vi "OuputMixer5782_1Ghz.vi"(6 "reset":bool, 8 "valid in":bool, 9 "Sine in":fxp<+/-,16,0>[](array[numeric])=[0.0, 0.0, 0.0, 0.0, 0.0, 0.0, 0.0, 0.0], 10 "Cosine in":fxp<+/-,16,0>[](array[numeric])=[0.0, 0.0, 0.0, 0.0, 0.0, 0.0, 0.0, 0.0], 11 "Data in":fxp<+/-,16,14>[](array[numeric])=[0.0, 0.0]) -> (0 "valid out":bool, 3 "test":i16[](array[numeric]))   [LabVIEW 2013]
doc: "Outputs input from channel 0 as I*cos(t)-Q*sin(t) on analog output 0"
uses:
  <vilib>/eio/EIONode/EIONode.xnode
  <vilib>/rvi/eio/common/nirviEmuTemplateMethod_errors.vi
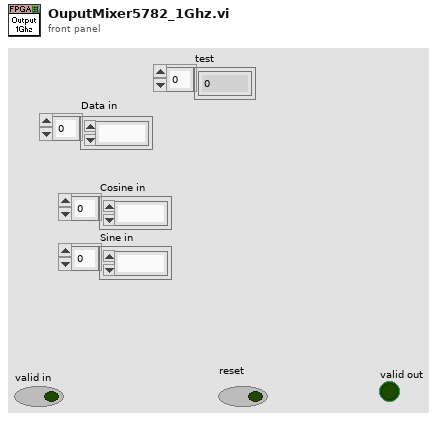
[diagram p1: front panel]
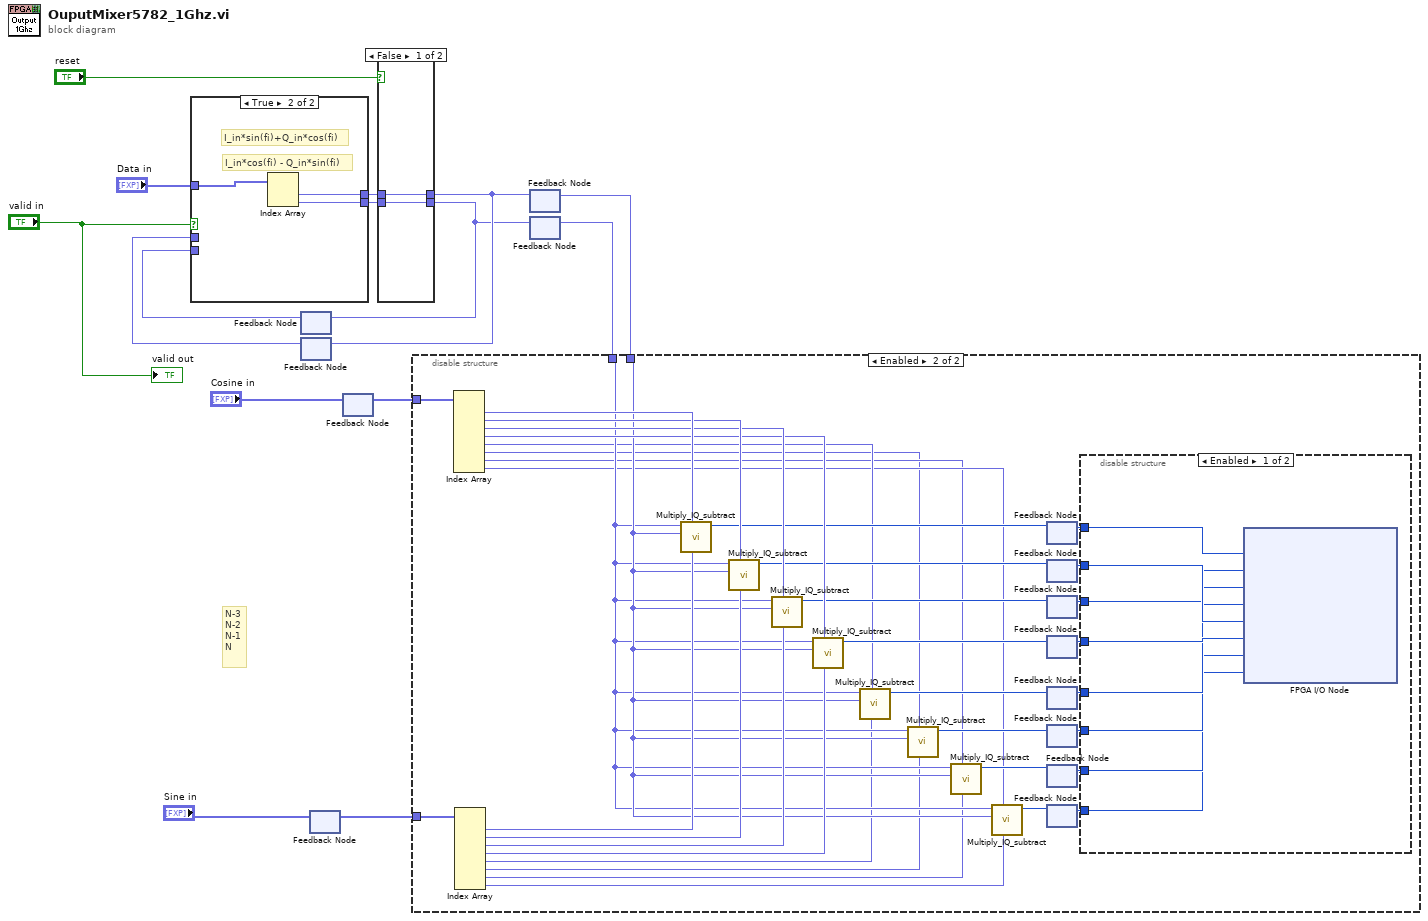
[diagram p0: block diagram]
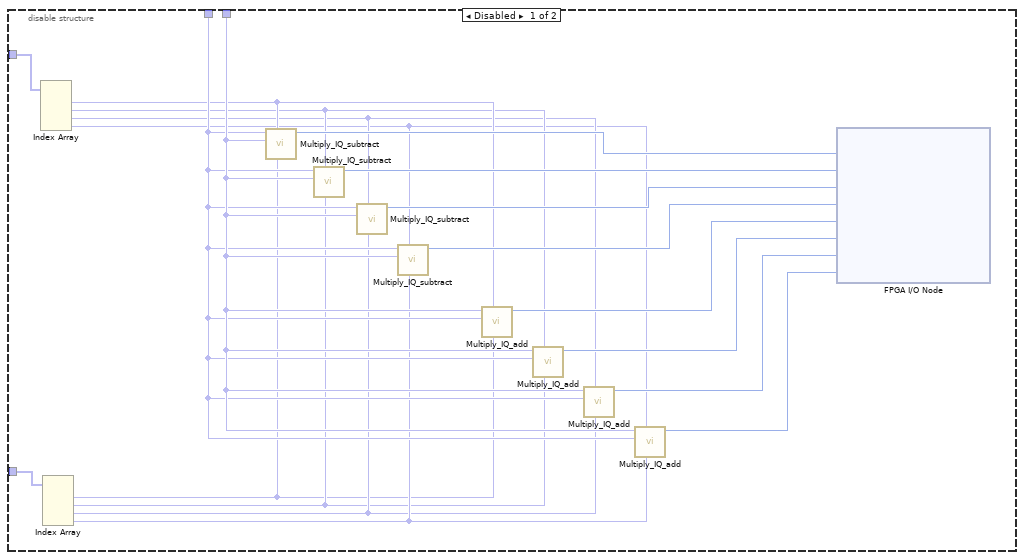
[diagram p2: hidden frame]
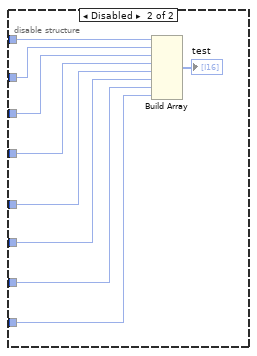
[diagram p3: hidden frame]
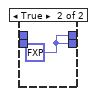
[diagram p4: hidden frame]
diagram:
  # "N-3\nN-2\nN-1\nN"
  n1 = feedback #1() -> (w12:fxp<+/-,16,14>)  [unwired: 1 in]
  n2 = feedback #2() -> (w11:fxp<+/-,16,14>)  [unwired: 1 in]
  n3 = case shown="True" "valid in" {
    tunnel: "Data in" -> [_ w20]
    tunnel: w12 -> [w16 _]
    tunnel: w11 -> [w17 _]
    tunnel: [w17 w19] -> w10
    tunnel: [w16 w18] -> w9
    frame False {
      # "keep old values"
    }
    frame True {
      # "I_in*cos(fi) - Q_in*sin(fi)"
      # "I_in*sin(fi)+Q_in*cos(fi)"
      n4 = Index Array(array=w20) -> (element #1=w19:fxp<+/-,16,14>, element #2=w18:fxp<+/-,16,14>)  [unwired: 2 in]
    }
  }
  n5 = feedback #3() -> (w8:fxp<+/-,16,0>[])  [unwired: 1 in]
  n6 = feedback-in #3("Sine in") -> ()
  n7 = feedback #4() -> (w7:fxp<+/-,16,0>[])  [unwired: 1 in]
  n8 = feedback-in #4("Cosine in") -> ()
  n9 = case shown="False" "reset" {
    tunnel: w10 -> [w21 _]
    tunnel: w9 -> [w22 _]
    tunnel: [w22 w23] -> w4
    tunnel: [w21 w23] -> w6
    frame False {
    }
    frame True {
      w23 = fxp<+/-,16,14> 0.0 ("Q in")
    }
  }
  n10 = feedback-in #1(w4) -> ()
  n11 = feedback-in #2(w6) -> ()
  n12 = feedback #5() -> (w5:fxp<+/-,16,14>)  [unwired: 1 in]
  n13 = feedback-in #5(w6) -> ()
  n14 = feedback #6() -> (w3:fxp<+/-,16,14>)  [unwired: 1 in]
  n15 = disable-structure shown="Enabled" {
    disable-tunnel: w5 -> [w39 w64]
    disable-tunnel: w3 -> [w38 w63]
    disable-tunnel: w7 -> [w33 w79]
    disable-tunnel: w8 -> [w32 w78]
    frame Disabled {
      n16 = Index Array(array=w33) -> (element #1=w31:fxp<+/-,16,0>, element #2=w30:fxp<+/-,16,0>, element #3=w29:fxp<+/-,16,0>, element #4=w28:fxp<+/-,16,0>)  [unwired: 4 in]
      n17 = Index Array(array=w32) -> (element #1=w24:fxp<+/-,16,0>, element #2=w25:fxp<+/-,16,0>, element #3=w26:fxp<+/-,16,0>, element #4=w27:fxp<+/-,16,0>)  [unwired: 4 in]
      n18 = call "Multiply_IQ_subtract.vi"("Sin"=w24, "Cos"=w31, "Q"=w39, "I"=w38) -> ("Z"=w43:i16)  [unwired: 6 in, 1 out]
      n19 = call "Multiply_IQ_subtract.vi"("Sin"=w25, "Cos"=w30, "Q"=w39, "I"=w38) -> ("Z"=w42:i16)  [unwired: 6 in, 1 out]
      n20 = call "Multiply_IQ_subtract.vi"("Sin"=w26, "Cos"=w29, "Q"=w39, "I"=w38) -> ("Z"=w41:i16)  [unwired: 6 in, 1 out]
      n21 = call "Multiply_IQ_subtract.vi"("Sin"=w27, "Cos"=w28, "Q"=w39, "I"=w38) -> ("Z"=w40:i16)  [unwired: 6 in, 1 out]
      n22 = call "Multiply_IQ_add.vi"("Sin"=w24, "Cos"=w31, "Q"=w38, "I"=w39) -> ("Z"=w37:i16)  [unwired: 6 in, 1 out]
      n23 = call "Multiply_IQ_add.vi"("Sin"=w25, "Cos"=w30, "Q"=w38, "I"=w39) -> ("Z"=w36:i16)  [unwired: 6 in, 1 out]
      n24 = call "Multiply_IQ_add.vi"("Sin"=w26, "Cos"=w29, "Q"=w38, "I"=w39) -> ("Z"=w35:i16)  [unwired: 6 in, 1 out]
      n25 = call "Multiply_IQ_add.vi"("Sin"=w27, "Cos"=w28, "Q"=w38, "I"=w39) -> ("Z"=w34:i16)  [unwired: 6 in, 1 out]
      n26 = xnode "FPGA I/O Node"("IO Module\\AO 0 N-3"=w43, "IO Module\\AO 0 N-2"=w42, "IO Module\\AO 0 N-1"=w41, "IO Module\\AO 0 N"=w40, "IO Module\\AO 1 N-3"=w37, "IO Module\\AO 1 N-2"=w36, "IO Module\\AO 1 N-1"=w35, "IO Module\\AO 1 N"=w34) -> ()  [unwired: 8 in, 8 out]
    }
    frame Enabled {
      n27 = Index Array(array=w79) -> (element #1=w77:fxp<+/-,16,0>, element #2=w76:fxp<+/-,16,0>, element #3=w75:fxp<+/-,16,0>, element #4=w74:fxp<+/-,16,0>, element #5=w54:fxp<+/-,16,0>, element #6=w51:fxp<+/-,16,0>, element #7=w52:fxp<+/-,16,0>, element #8=w53:fxp<+/-,16,0>)  [unwired: 8 in]
      n28 = Index Array(array=w78) -> (element #1=w70:fxp<+/-,16,0>, element #2=w71:fxp<+/-,16,0>, element #3=w72:fxp<+/-,16,0>, element #4=w73:fxp<+/-,16,0>, element #5=w62:fxp<+/-,16,0>, element #6=w61:fxp<+/-,16,0>, element #7=w60:fxp<+/-,16,0>, element #8=w59:fxp<+/-,16,0>)  [unwired: 8 in]
      n29 = call "Multiply_IQ_subtract.vi"("Sin"=w70, "Cos"=w77, "Q"=w64, "I"=w63) -> ("Z"=w69:i16)  [unwired: 6 in, 1 out]
      n30 = call "Multiply_IQ_subtract.vi"("Sin"=w71, "Cos"=w76, "Q"=w64, "I"=w63) -> ("Z"=w68:i16)  [unwired: 6 in, 1 out]
      n31 = call "Multiply_IQ_subtract.vi"("Sin"=w72, "Cos"=w75, "Q"=w64, "I"=w63) -> ("Z"=w67:i16)  [unwired: 6 in, 1 out]
      n32 = call "Multiply_IQ_subtract.vi"("Sin"=w73, "Cos"=w74, "Q"=w64, "I"=w63) -> ("Z"=w66:i16)  [unwired: 6 in, 1 out]
      n33 = call "Multiply_IQ_subtract.vi"("Sin"=w62, "Cos"=w54, "Q"=w64, "I"=w63) -> ("Z"=w58:i16)  [unwired: 6 in, 1 out]
      n34 = call "Multiply_IQ_subtract.vi"("Sin"=w61, "Cos"=w51, "Q"=w64, "I"=w63) -> ("Z"=w57:i16)  [unwired: 6 in, 1 out]
      n35 = call "Multiply_IQ_subtract.vi"("Sin"=w60, "Cos"=w52, "Q"=w64, "I"=w63) -> ("Z"=w56:i16)  [unwired: 6 in, 1 out]
      n36 = call "Multiply_IQ_subtract.vi"("Sin"=w59, "Cos"=w53, "Q"=w64, "I"=w63) -> ("Z"=w55:i16)  [unwired: 6 in, 1 out]
      n37 = feedback #7() -> (w65:i16)  [unwired: 1 in]
      n38 = feedback-in #7(w69) -> ()
      n39 = feedback #8() -> (w50:i16)  [unwired: 1 in]
      n40 = feedback-in #8(w68) -> ()
      n41 = feedback #9() -> (w49:i16)  [unwired: 1 in]
      n42 = feedback-in #9(w67) -> ()
      n43 = feedback #10() -> (w48:i16)  [unwired: 1 in]
      n44 = feedback-in #10(w66) -> ()
      n45 = feedback #11() -> (w47:i16)  [unwired: 1 in]
      n46 = feedback-in #11(w58) -> ()
      n47 = feedback #12() -> (w46:i16)  [unwired: 1 in]
      n48 = feedback-in #12(w57) -> ()
      n49 = feedback #13() -> (w45:i16)  [unwired: 1 in]
      n50 = feedback-in #13(w56) -> ()
      n51 = feedback #14() -> (w44:i16)  [unwired: 1 in]
      n52 = feedback-in #14(w55) -> ()
      n53 = disable-structure shown="Enabled" {
        disable-tunnel: w65 -> [w87 w96]
        disable-tunnel: w50 -> [w86 w95]
        disable-tunnel: w49 -> [w85 w94]
        disable-tunnel: w48 -> [w84 w93]
        disable-tunnel: w47 -> [w83 w92]
        disable-tunnel: w46 -> [w82 w91]
        disable-tunnel: w45 -> [w81 w90]
        disable-tunnel: w44 -> [w80 w89]
        frame Enabled {
          n54 = xnode "FPGA I/O Node"("IO Module\\AO 0 N-3"=w87, "IO Module\\AO 0 N-2"=w85, "IO Module\\AO 0 N-1"=w83, "IO Module\\AO 0 N"=w81, "IO Module\\AO 1 N-3"=w86, "IO Module\\AO 1 N-2"=w84, "IO Module\\AO 1 N-1"=w82, "IO Module\\AO 1 N"=w80) -> ()  [unwired: 8 in, 8 out]
        }
        frame Disabled {
          n55 = Build Array(w96, w95, w94, w93, w92, w91, w90, w89) -> (→"test":i16[])
        }
      }
    }
  }
  n56 = feedback-in #6(w4) -> ()
  "valid out" <- "valid in"
